vi "old LED STATUS for BLINKIN.vi"() -> ()   [LabVIEW 2023]
uses:
  ctrl defs/ctrl LED STATES.ctl
  <vilib>/Rock Robotics/WPI/DriverStation/WPI_DriverStationRobotMode2.ctl
  <vilib>/Rock Robotics/WPI/DriverStation/WPI_DriverStationAllianceInfo.ctl
  ctrl defs/ctrl LED PATTERNS.ctl
  Global INIT.vi
  Global stack names.vi
  <vilib>/Rock Robotics/Network Tables/NT Read Boolean.vi
  Global odometry.vi
panel:
  in  "ARMS LOCKED":T1=22 items=["<<Select a pattern>>", "Rainbow, Rainbow palette", "Rainbow, Party palette", "Rainbow, Ocean palette", "Rainbow, Lava palette", "Rainbow, Forest palette", "Rainbow with glitter", "Confetti", "Shot, Red", "Shot, Blue", "Shot, White", "Sinelon, Rainbow palette", "Sinelon, Party palette", "Sinelon, Ocean palette", "Sinelon, Lava palette", "Sinelon, Forest palette", "BPM, Rainbow palette", "BPM, Party palette", "BPM, Ocean palette", "BPM, Lava palette", "BPM, Forest palette", "Fire, Medium", "Fire, Large", "Twinkles, Rainbow palette", "Twinkles, Party palette", "Twinkles, Ocean palette", "Twinkles, Lava palette", "Twinkles, Forest palette", "Color Waves, Rainbow palette", "Color Waves, Party palette", "Color Waves, Ocean palette", "Color Waves, Lava palette", "Color Waves, Forest palette", "Larson Scanner, Red", "Larson Scanner, Gray", "Light Chase, Red", "Light Chase, Blue", "Light Chase, Gray", "Heartbeat, Red", "Heartbeat, Blue", "Heartbeat, White", "Heartbeat, Gray", "Breath, Red", "Breath, Blue", "Breath, Gray", "Strobe, Red", "Strobe, Blue", "Strobe, Gold", "Strobe, White", "Color 1: End to End Blend to Black", "Color 1: Larson Scanner", "Color 1: Light Chase", "Color 1: Heartbeat Slow", "Color 1: Heartbeat Medium", "Color 1: Heartbeat Fast", "Color 1: Breath Slow", "Color 1: Breath Fast", "Color 1: Shot", "Color 1: Strobe", "Color 2: End to End Blend to Black", "Color 2: Larson Scanner", "Color 2: Light Chase", "Color 2: Heartbeat Slow", "Color 2: Heartbeat Medium", "Color 2: Heartbeat Fast", "Color 2: Breath Slow", "Color 2: Breath Fast", "Color 2: Shot", "Color 2: Strobe", "Color 1/2: Sparkle, 1 on 2", "Color 1/2: Sparkle 2 on 1", "Color 1/2: Gradient", "Color 1/2: BPM", "Color 1/2: End to End Blend 1 to 2", "Color 1/2: End to End Blend 2 to 1", "Color 1/2: setup pattern", "Color 1/2: Twinkles", "Color 1/2: Color Waves", "Color 1/2: Sinelon", "Solid Hot Pink", "Solid Dark Red", "Solid Red", "Solid Red Orange", "Solid Orange", "Solid Gold", "Solid Yellow", "Solid Lawn Green", "Solid Lime", "Solid Dark Green", "Solid Green", "Solid Blue Green", "Solid Aqua", "Solid Sky Blue", "Solid Dark Blue", "Solid Blue", "Solid Blue Violet", "Solid Violet", "Solid White", "Solid Gray", "Solid Dark Gray", "Solid Black"]
  in  "PUKE":T1=79 items=["<<Select a pattern>>", "Rainbow, Rainbow palette", "Rainbow, Party palette", "Rainbow, Ocean palette", "Rainbow, Lava palette", "Rainbow, Forest palette", "Rainbow with glitter", "Confetti", "Shot, Red", "Shot, Blue", "Shot, White", "Sinelon, Rainbow palette", "Sinelon, Party palette", "Sinelon, Ocean palette", "Sinelon, Lava palette", "Sinelon, Forest palette", "BPM, Rainbow palette", "BPM, Party palette", "BPM, Ocean palette", "BPM, Lava palette", "BPM, Forest palette", "Fire, Medium", "Fire, Large", "Twinkles, Rainbow palette", "Twinkles, Party palette", "Twinkles, Ocean palette", "Twinkles, Lava palette", "Twinkles, Forest palette", "Color Waves, Rainbow palette", "Color Waves, Party palette", "Color Waves, Ocean palette", "Color Waves, Lava palette", "Color Waves, Forest palette", "Larson Scanner, Red", "Larson Scanner, Gray", "Light Chase, Red", "Light Chase, Blue", "Light Chase, Gray", "Heartbeat, Red", "Heartbeat, Blue", "Heartbeat, White", "Heartbeat, Gray", "Breath, Red", "Breath, Blue", "Breath, Gray", "Strobe, Red", "Strobe, Blue", "Strobe, Gold", "Strobe, White", "Color 1: End to End Blend to Black", "Color 1: Larson Scanner", "Color 1: Light Chase", "Color 1: Heartbeat Slow", "Color 1: Heartbeat Medium", "Color 1: Heartbeat Fast", "Color 1: Breath Slow", "Color 1: Breath Fast", "Color 1: Shot", "Color 1: Strobe", "Color 2: End to End Blend to Black", "Color 2: Larson Scanner", "Color 2: Light Chase", "Color 2: Heartbeat Slow", "Color 2: Heartbeat Medium", "Color 2: Heartbeat Fast", "Color 2: Breath Slow", "Color 2: Breath Fast", "Color 2: Shot", "Color 2: Strobe", "Color 1/2: Sparkle, 1 on 2", "Color 1/2: Sparkle 2 on 1", "Color 1/2: Gradient", "Color 1/2: BPM", "Color 1/2: End to End Blend 1 to 2", "Color 1/2: End to End Blend 2 to 1", "Color 1/2: setup pattern", "Color 1/2: Twinkles", "Color 1/2: Color Waves", "Color 1/2: Sinelon", "Solid Hot Pink", "Solid Dark Red", "Solid Red", "Solid Red Orange", "Solid Orange", "Solid Gold", "Solid Yellow", "Solid Lawn Green", "Solid Lime", "Solid Dark Green", "Solid Green", "Solid Blue Green", "Solid Aqua", "Solid Sky Blue", "Solid Dark Blue", "Solid Blue", "Solid Blue Violet", "Solid Violet", "Solid White", "Solid Gray", "Solid Dark Gray", "Solid Black"]
  in  "LOOKING for NOTE":T1=33 items=["<<Select a pattern>>", "Rainbow, Rainbow palette", "Rainbow, Party palette", "Rainbow, Ocean palette", "Rainbow, Lava palette", "Rainbow, Forest palette", "Rainbow with glitter", "Confetti", "Shot, Red", "Shot, Blue", "Shot, White", "Sinelon, Rainbow palette", "Sinelon, Party palette", "Sinelon, Ocean palette", "Sinelon, Lava palette", "Sinelon, Forest palette", "BPM, Rainbow palette", "BPM, Party palette", "BPM, Ocean palette", "BPM, Lava palette", "BPM, Forest palette", "Fire, Medium", "Fire, Large", "Twinkles, Rainbow palette", "Twinkles, Party palette", "Twinkles, Ocean palette", "Twinkles, Lava palette", "Twinkles, Forest palette", "Color Waves, Rainbow palette", "Color Waves, Party palette", "Color Waves, Ocean palette", "Color Waves, Lava palette", "Color Waves, Forest palette", "Larson Scanner, Red", "Larson Scanner, Gray", "Light Chase, Red", "Light Chase, Blue", "Light Chase, Gray", "Heartbeat, Red", "Heartbeat, Blue", "Heartbeat, White", "Heartbeat, Gray", "Breath, Red", "Breath, Blue", "Breath, Gray", "Strobe, Red", "Strobe, Blue", "Strobe, Gold", "Strobe, White", "Color 1: End to End Blend to Black", "Color 1: Larson Scanner", "Color 1: Light Chase", "Color 1: Heartbeat Slow", "Color 1: Heartbeat Medium", "Color 1: Heartbeat Fast", "Color 1: Breath Slow", "Color 1: Breath Fast", "Color 1: Shot", "Color 1: Strobe", "Color 2: End to End Blend to Black", "Color 2: Larson Scanner", "Color 2: Light Chase", "Color 2: Heartbeat Slow", "Color 2: Heartbeat Medium", "Color 2: Heartbeat Fast", "Color 2: Breath Slow", "Color 2: Breath Fast", "Color 2: Shot", "Color 2: Strobe", "Color 1/2: Sparkle, 1 on 2", "Color 1/2: Sparkle 2 on 1", "Color 1/2: Gradient", "Color 1/2: BPM", "Color 1/2: End to End Blend 1 to 2", "Color 1/2: End to End Blend 2 to 1", "Color 1/2: setup pattern", "Color 1/2: Twinkles", "Color 1/2: Color Waves", "Color 1/2: Sinelon", "Solid Hot Pink", "Solid Dark Red", "Solid Red", "Solid Red Orange", "Solid Orange", "Solid Gold", "Solid Yellow", "Solid Lawn Green", "Solid Lime", "Solid Dark Green", "Solid Green", "Solid Blue Green", "Solid Aqua", "Solid Sky Blue", "Solid Dark Blue", "Solid Blue", "Solid Blue Violet", "Solid Violet", "Solid White", "Solid Gray", "Solid Dark Gray", "Solid Black"]
  in  "NOTE LOADED":T1=89 items=["<<Select a pattern>>", "Rainbow, Rainbow palette", "Rainbow, Party palette", "Rainbow, Ocean palette", "Rainbow, Lava palette", "Rainbow, Forest palette", "Rainbow with glitter", "Confetti", "Shot, Red", "Shot, Blue", "Shot, White", "Sinelon, Rainbow palette", "Sinelon, Party palette", "Sinelon, Ocean palette", "Sinelon, Lava palette", "Sinelon, Forest palette", "BPM, Rainbow palette", "BPM, Party palette", "BPM, Ocean palette", "BPM, Lava palette", "BPM, Forest palette", "Fire, Medium", "Fire, Large", "Twinkles, Rainbow palette", "Twinkles, Party palette", "Twinkles, Ocean palette", "Twinkles, Lava palette", "Twinkles, Forest palette", "Color Waves, Rainbow palette", "Color Waves, Party palette", "Color Waves, Ocean palette", "Color Waves, Lava palette", "Color Waves, Forest palette", "Larson Scanner, Red", "Larson Scanner, Gray", "Light Chase, Red", "Light Chase, Blue", "Light Chase, Gray", "Heartbeat, Red", "Heartbeat, Blue", "Heartbeat, White", "Heartbeat, Gray", "Breath, Red", "Breath, Blue", "Breath, Gray", "Strobe, Red", "Strobe, Blue", "Strobe, Gold", "Strobe, White", "Color 1: End to End Blend to Black", "Color 1: Larson Scanner", "Color 1: Light Chase", "Color 1: Heartbeat Slow", "Color 1: Heartbeat Medium", "Color 1: Heartbeat Fast", "Color 1: Breath Slow", "Color 1: Breath Fast", "Color 1: Shot", "Color 1: Strobe", "Color 2: End to End Blend to Black", "Color 2: Larson Scanner", "Color 2: Light Chase", "Color 2: Heartbeat Slow", "Color 2: Heartbeat Medium", "Color 2: Heartbeat Fast", "Color 2: Breath Slow", "Color 2: Breath Fast", "Color 2: Shot", "Color 2: Strobe", "Color 1/2: Sparkle, 1 on 2", "Color 1/2: Sparkle 2 on 1", "Color 1/2: Gradient", "Color 1/2: BPM", "Color 1/2: End to End Blend 1 to 2", "Color 1/2: End to End Blend 2 to 1", "Color 1/2: setup pattern", "Color 1/2: Twinkles", "Color 1/2: Color Waves", "Color 1/2: Sinelon", "Solid Hot Pink", "Solid Dark Red", "Solid Red", "Solid Red Orange", "Solid Orange", "Solid Gold", "Solid Yellow", "Solid Lawn Green", "Solid Lime", "Solid Dark Green", "Solid Green", "Solid Blue Green", "Solid Aqua", "Solid Sky Blue", "Solid Dark Blue", "Solid Blue", "Solid Blue Violet", "Solid Violet", "Solid White", "Solid Gray", "Solid Dark Gray", "Solid Black"]
  in  "END GAME 2":T1=94 items=["<<Select a pattern>>", "Rainbow, Rainbow palette", "Rainbow, Party palette", "Rainbow, Ocean palette", "Rainbow, Lava palette", "Rainbow, Forest palette", "Rainbow with glitter", "Confetti", "Shot, Red", "Shot, Blue", "Shot, White", "Sinelon, Rainbow palette", "Sinelon, Party palette", "Sinelon, Ocean palette", "Sinelon, Lava palette", "Sinelon, Forest palette", "BPM, Rainbow palette", "BPM, Party palette", "BPM, Ocean palette", "BPM, Lava palette", "BPM, Forest palette", "Fire, Medium", "Fire, Large", "Twinkles, Rainbow palette", "Twinkles, Party palette", "Twinkles, Ocean palette", "Twinkles, Lava palette", "Twinkles, Forest palette", "Color Waves, Rainbow palette", "Color Waves, Party palette", "Color Waves, Ocean palette", "Color Waves, Lava palette", "Color Waves, Forest palette", "Larson Scanner, Red", "Larson Scanner, Gray", "Light Chase, Red", "Light Chase, Blue", "Light Chase, Gray", "Heartbeat, Red", "Heartbeat, Blue", "Heartbeat, White", "Heartbeat, Gray", "Breath, Red", "Breath, Blue", "Breath, Gray", "Strobe, Red", "Strobe, Blue", "Strobe, Gold", "Strobe, White", "Color 1: End to End Blend to Black", "Color 1: Larson Scanner", "Color 1: Light Chase", "Color 1: Heartbeat Slow", "Color 1: Heartbeat Medium", "Color 1: Heartbeat Fast", "Color 1: Breath Slow", "Color 1: Breath Fast", "Color 1: Shot", "Color 1: Strobe", "Color 2: End to End Blend to Black", "Color 2: Larson Scanner", "Color 2: Light Chase", "Color 2: Heartbeat Slow", "Color 2: Heartbeat Medium", "Color 2: Heartbeat Fast", "Color 2: Breath Slow", "Color 2: Breath Fast", "Color 2: Shot", "Color 2: Strobe", "Color 1/2: Sparkle, 1 on 2", "Color 1/2: Sparkle 2 on 1", "Color 1/2: Gradient", "Color 1/2: BPM", "Color 1/2: End to End Blend 1 to 2", "Color 1/2: End to End Blend 2 to 1", "Color 1/2: setup pattern", "Color 1/2: Twinkles", "Color 1/2: Color Waves", "Color 1/2: Sinelon", "Solid Hot Pink", "Solid Dark Red", "Solid Red", "Solid Red Orange", "Solid Orange", "Solid Gold", "Solid Yellow", "Solid Lawn Green", "Solid Lime", "Solid Dark Green", "Solid Green", "Solid Blue Green", "Solid Aqua", "Solid Sky Blue", "Solid Dark Blue", "Solid Blue", "Solid Blue Violet", "Solid Violet", "Solid White", "Solid Gray", "Solid Dark Gray", "Solid Black"]
  in  "END GAME 1":T1=85 items=["<<Select a pattern>>", "Rainbow, Rainbow palette", "Rainbow, Party palette", "Rainbow, Ocean palette", "Rainbow, Lava palette", "Rainbow, Forest palette", "Rainbow with glitter", "Confetti", "Shot, Red", "Shot, Blue", "Shot, White", "Sinelon, Rainbow palette", "Sinelon, Party palette", "Sinelon, Ocean palette", "Sinelon, Lava palette", "Sinelon, Forest palette", "BPM, Rainbow palette", "BPM, Party palette", "BPM, Ocean palette", "BPM, Lava palette", "BPM, Forest palette", "Fire, Medium", "Fire, Large", "Twinkles, Rainbow palette", "Twinkles, Party palette", "Twinkles, Ocean palette", "Twinkles, Lava palette", "Twinkles, Forest palette", "Color Waves, Rainbow palette", "Color Waves, Party palette", "Color Waves, Ocean palette", "Color Waves, Lava palette", "Color Waves, Forest palette", "Larson Scanner, Red", "Larson Scanner, Gray", "Light Chase, Red", "Light Chase, Blue", "Light Chase, Gray", "Heartbeat, Red", "Heartbeat, Blue", "Heartbeat, White", "Heartbeat, Gray", "Breath, Red", "Breath, Blue", "Breath, Gray", "Strobe, Red", "Strobe, Blue", "Strobe, Gold", "Strobe, White", "Color 1: End to End Blend to Black", "Color 1: Larson Scanner", "Color 1: Light Chase", "Color 1: Heartbeat Slow", "Color 1: Heartbeat Medium", "Color 1: Heartbeat Fast", "Color 1: Breath Slow", "Color 1: Breath Fast", "Color 1: Shot", "Color 1: Strobe", "Color 2: End to End Blend to Black", "Color 2: Larson Scanner", "Color 2: Light Chase", "Color 2: Heartbeat Slow", "Color 2: Heartbeat Medium", "Color 2: Heartbeat Fast", "Color 2: Breath Slow", "Color 2: Breath Fast", "Color 2: Shot", "Color 2: Strobe", "Color 1/2: Sparkle, 1 on 2", "Color 1/2: Sparkle 2 on 1", "Color 1/2: Gradient", "Color 1/2: BPM", "Color 1/2: End to End Blend 1 to 2", "Color 1/2: End to End Blend 2 to 1", "Color 1/2: setup pattern", "Color 1/2: Twinkles", "Color 1/2: Color Waves", "Color 1/2: Sinelon", "Solid Hot Pink", "Solid Dark Red", "Solid Red", "Solid Red Orange", "Solid Orange", "Solid Gold", "Solid Yellow", "Solid Lawn Green", "Solid Lime", "Solid Dark Green", "Solid Green", "Solid Blue Green", "Solid Aqua", "Solid Sky Blue", "Solid Dark Blue", "Solid Blue", "Solid Blue Violet", "Solid Violet", "Solid White", "Solid Gray", "Solid Dark Gray", "Solid Black"]
  in  "LOW BATT":T1=45 items=["<<Select a pattern>>", "Rainbow, Rainbow palette", "Rainbow, Party palette", "Rainbow, Ocean palette", "Rainbow, Lava palette", "Rainbow, Forest palette", "Rainbow with glitter", "Confetti", "Shot, Red", "Shot, Blue", "Shot, White", "Sinelon, Rainbow palette", "Sinelon, Party palette", "Sinelon, Ocean palette", "Sinelon, Lava palette", "Sinelon, Forest palette", "BPM, Rainbow palette", "BPM, Party palette", "BPM, Ocean palette", "BPM, Lava palette", "BPM, Forest palette", "Fire, Medium", "Fire, Large", "Twinkles, Rainbow palette", "Twinkles, Party palette", "Twinkles, Ocean palette", "Twinkles, Lava palette", "Twinkles, Forest palette", "Color Waves, Rainbow palette", "Color Waves, Party palette", "Color Waves, Ocean palette", "Color Waves, Lava palette", "Color Waves, Forest palette", "Larson Scanner, Red", "Larson Scanner, Gray", "Light Chase, Red", "Light Chase, Blue", "Light Chase, Gray", "Heartbeat, Red", "Heartbeat, Blue", "Heartbeat, White", "Heartbeat, Gray", "Breath, Red", "Breath, Blue", "Breath, Gray", "Strobe, Red", "Strobe, Blue", "Strobe, Gold", "Strobe, White", "Color 1: End to End Blend to Black", "Color 1: Larson Scanner", "Color 1: Light Chase", "Color 1: Heartbeat Slow", "Color 1: Heartbeat Medium", "Color 1: Heartbeat Fast", "Color 1: Breath Slow", "Color 1: Breath Fast", "Color 1: Shot", "Color 1: Strobe", "Color 2: End to End Blend to Black", "Color 2: Larson Scanner", "Color 2: Light Chase", "Color 2: Heartbeat Slow", "Color 2: Heartbeat Medium", "Color 2: Heartbeat Fast", "Color 2: Breath Slow", "Color 2: Breath Fast", "Color 2: Shot", "Color 2: Strobe", "Color 1/2: Sparkle, 1 on 2", "Color 1/2: Sparkle 2 on 1", "Color 1/2: Gradient", "Color 1/2: BPM", "Color 1/2: End to End Blend 1 to 2", "Color 1/2: End to End Blend 2 to 1", "Color 1/2: setup pattern", "Color 1/2: Twinkles", "Color 1/2: Color Waves", "Color 1/2: Sinelon", "Solid Hot Pink", "Solid Dark Red", "Solid Red", "Solid Red Orange", "Solid Orange", "Solid Gold", "Solid Yellow", "Solid Lawn Green", "Solid Lime", "Solid Dark Green", "Solid Green", "Solid Blue Green", "Solid Aqua", "Solid Sky Blue", "Solid Dark Blue", "Solid Blue", "Solid Blue Violet", "Solid Violet", "Solid White", "Solid Gray", "Solid Dark Gray", "Solid Black"]
  in  "SELECT  AMP":T1=47 items=["<<Select a pattern>>", "Rainbow, Rainbow palette", "Rainbow, Party palette", "Rainbow, Ocean palette", "Rainbow, Lava palette", "Rainbow, Forest palette", "Rainbow with glitter", "Confetti", "Shot, Red", "Shot, Blue", "Shot, White", "Sinelon, Rainbow palette", "Sinelon, Party palette", "Sinelon, Ocean palette", "Sinelon, Lava palette", "Sinelon, Forest palette", "BPM, Rainbow palette", "BPM, Party palette", "BPM, Ocean palette", "BPM, Lava palette", "BPM, Forest palette", "Fire, Medium", "Fire, Large", "Twinkles, Rainbow palette", "Twinkles, Party palette", "Twinkles, Ocean palette", "Twinkles, Lava palette", "Twinkles, Forest palette", "Color Waves, Rainbow palette", "Color Waves, Party palette", "Color Waves, Ocean palette", "Color Waves, Lava palette", "Color Waves, Forest palette", "Larson Scanner, Red", "Larson Scanner, Gray", "Light Chase, Red", "Light Chase, Blue", "Light Chase, Gray", "Heartbeat, Red", "Heartbeat, Blue", "Heartbeat, White", "Heartbeat, Gray", "Breath, Red", "Breath, Blue", "Breath, Gray", "Strobe, Red", "Strobe, Blue", "Strobe, Gold", "Strobe, White", "Color 1: End to End Blend to Black", "Color 1: Larson Scanner", "Color 1: Light Chase", "Color 1: Heartbeat Slow", "Color 1: Heartbeat Medium", "Color 1: Heartbeat Fast", "Color 1: Breath Slow", "Color 1: Breath Fast", "Color 1: Shot", "Color 1: Strobe", "Color 2: End to End Blend to Black", "Color 2: Larson Scanner", "Color 2: Light Chase", "Color 2: Heartbeat Slow", "Color 2: Heartbeat Medium", "Color 2: Heartbeat Fast", "Color 2: Breath Slow", "Color 2: Breath Fast", "Color 2: Shot", "Color 2: Strobe", "Color 1/2: Sparkle, 1 on 2", "Color 1/2: Sparkle 2 on 1", "Color 1/2: Gradient", "Color 1/2: BPM", "Color 1/2: End to End Blend 1 to 2", "Color 1/2: End to End Blend 2 to 1", "Color 1/2: setup pattern", "Color 1/2: Twinkles", "Color 1/2: Color Waves", "Color 1/2: Sinelon", "Solid Hot Pink", "Solid Dark Red", "Solid Red", "Solid Red Orange", "Solid Orange", "Solid Gold", "Solid Yellow", "Solid Lawn Green", "Solid Lime", "Solid Dark Green", "Solid Green", "Solid Blue Green", "Solid Aqua", "Solid Sky Blue", "Solid Dark Blue", "Solid Blue", "Solid Blue Violet", "Solid Violet", "Solid White", "Solid Gray", "Solid Dark Gray", "Solid Black"]
  in  "FIRE":T1=84 items=["<<Select a pattern>>", "Rainbow, Rainbow palette", "Rainbow, Party palette", "Rainbow, Ocean palette", "Rainbow, Lava palette", "Rainbow, Forest palette", "Rainbow with glitter", "Confetti", "Shot, Red", "Shot, Blue", "Shot, White", "Sinelon, Rainbow palette", "Sinelon, Party palette", "Sinelon, Ocean palette", "Sinelon, Lava palette", "Sinelon, Forest palette", "BPM, Rainbow palette", "BPM, Party palette", "BPM, Ocean palette", "BPM, Lava palette", "BPM, Forest palette", "Fire, Medium", "Fire, Large", "Twinkles, Rainbow palette", "Twinkles, Party palette", "Twinkles, Ocean palette", "Twinkles, Lava palette", "Twinkles, Forest palette", "Color Waves, Rainbow palette", "Color Waves, Party palette", "Color Waves, Ocean palette", "Color Waves, Lava palette", "Color Waves, Forest palette", "Larson Scanner, Red", "Larson Scanner, Gray", "Light Chase, Red", "Light Chase, Blue", "Light Chase, Gray", "Heartbeat, Red", "Heartbeat, Blue", "Heartbeat, White", "Heartbeat, Gray", "Breath, Red", "Breath, Blue", "Breath, Gray", "Strobe, Red", "Strobe, Blue", "Strobe, Gold", "Strobe, White", "Color 1: End to End Blend to Black", "Color 1: Larson Scanner", "Color 1: Light Chase", "Color 1: Heartbeat Slow", "Color 1: Heartbeat Medium", "Color 1: Heartbeat Fast", "Color 1: Breath Slow", "Color 1: Breath Fast", "Color 1: Shot", "Color 1: Strobe", "Color 2: End to End Blend to Black", "Color 2: Larson Scanner", "Color 2: Light Chase", "Color 2: Heartbeat Slow", "Color 2: Heartbeat Medium", "Color 2: Heartbeat Fast", "Color 2: Breath Slow", "Color 2: Breath Fast", "Color 2: Shot", "Color 2: Strobe", "Color 1/2: Sparkle, 1 on 2", "Color 1/2: Sparkle 2 on 1", "Color 1/2: Gradient", "Color 1/2: BPM", "Color 1/2: End to End Blend 1 to 2", "Color 1/2: End to End Blend 2 to 1", "Color 1/2: setup pattern", "Color 1/2: Twinkles", "Color 1/2: Color Waves", "Color 1/2: Sinelon", "Solid Hot Pink", "Solid Dark Red", "Solid Red", "Solid Red Orange", "Solid Orange", "Solid Gold", "Solid Yellow", "Solid Lawn Green", "Solid Lime", "Solid Dark Green", "Solid Green", "Solid Blue Green", "Solid Aqua", "Solid Sky Blue", "Solid Dark Blue", "Solid Blue", "Solid Blue Violet", "Solid Violet", "Solid White", "Solid Gray", "Solid Dark Gray", "Solid Black"]
  in  "DEFAULT":T1=75 items=["<<Select a pattern>>", "Rainbow, Rainbow palette", "Rainbow, Party palette", "Rainbow, Ocean palette", "Rainbow, Lava palette", "Rainbow, Forest palette", "Rainbow with glitter", "Confetti", "Shot, Red", "Shot, Blue", "Shot, White", "Sinelon, Rainbow palette", "Sinelon, Party palette", "Sinelon, Ocean palette", "Sinelon, Lava palette", "Sinelon, Forest palette", "BPM, Rainbow palette", "BPM, Party palette", "BPM, Ocean palette", "BPM, Lava palette", "BPM, Forest palette", "Fire, Medium", "Fire, Large", "Twinkles, Rainbow palette", "Twinkles, Party palette", "Twinkles, Ocean palette", "Twinkles, Lava palette", "Twinkles, Forest palette", "Color Waves, Rainbow palette", "Color Waves, Party palette", "Color Waves, Ocean palette", "Color Waves, Lava palette", "Color Waves, Forest palette", "Larson Scanner, Red", "Larson Scanner, Gray", "Light Chase, Red", "Light Chase, Blue", "Light Chase, Gray", "Heartbeat, Red", "Heartbeat, Blue", "Heartbeat, White", "Heartbeat, Gray", "Breath, Red", "Breath, Blue", "Breath, Gray", "Strobe, Red", "Strobe, Blue", "Strobe, Gold", "Strobe, White", "Color 1: End to End Blend to Black", "Color 1: Larson Scanner", "Color 1: Light Chase", "Color 1: Heartbeat Slow", "Color 1: Heartbeat Medium", "Color 1: Heartbeat Fast", "Color 1: Breath Slow", "Color 1: Breath Fast", "Color 1: Shot", "Color 1: Strobe", "Color 2: End to End Blend to Black", "Color 2: Larson Scanner", "Color 2: Light Chase", "Color 2: Heartbeat Slow", "Color 2: Heartbeat Medium", "Color 2: Heartbeat Fast", "Color 2: Breath Slow", "Color 2: Breath Fast", "Color 2: Shot", "Color 2: Strobe", "Color 1/2: Sparkle, 1 on 2", "Color 1/2: Sparkle 2 on 1", "Color 1/2: Gradient", "Color 1/2: BPM", "Color 1/2: End to End Blend 1 to 2", "Color 1/2: End to End Blend 2 to 1", "Color 1/2: setup pattern", "Color 1/2: Twinkles", "Color 1/2: Color Waves", "Color 1/2: Sinelon", "Solid Hot Pink", "Solid Dark Red", "Solid Red", "Solid Red Orange", "Solid Orange", "Solid Gold", "Solid Yellow", "Solid Lawn Green", "Solid Lime", "Solid Dark Green", "Solid Green", "Solid Blue Green", "Solid Aqua", "Solid Sky Blue", "Solid Dark Blue", "Solid Blue", "Solid Blue Violet", "Solid Violet", "Solid White", "Solid Gray", "Solid Dark Gray", "Solid Black"]
  out "Teleop indicators":T2
  out "Motor Output":dbl=0.49
  out "String":string="1 - Rainbow, Rainbow Palette\n2 - Rainbow, Party Palette\n3 - Rainbow, Ocean Palette\n4 - Rainbow, Lave Palette\n5 - Rainbow, Forest Palette\n6 - Rainbow with Glitter\n7 - Confetti\n8 - Shot, Red\n9 - Shot, Blue\n10 - Shot, White\n11 - Sinelon, Rainbow Palette\n12 - Sinelon, Party Palette\n13 - Sinelon, Ocean Palette\n14 - Sinelon, Lava Palette\n15 - Sinelon, Forest Palette\n16 - Beats per Minute, Rainbow Palette\n17 - Beats per Minute, Party Palette\n18 - Beats per Minute, Ocean Palette\n19 - Beats per Minute, Lava Palette\n20 - Beats per Minute, Forest Palette\n21 - Fire, Medium\n22 - Fire, Large\n23 - Twinkles, Rainbow Palette\n24 - Twinkles, Party Palette\n25 - Twinkles, Ocean Palette\n26 - Twinkles, Lava Palette\n27 - Twinkles, Forest Palette\n28 - Color Waves, Rainbow Palette\n29 - Color Waves, Party Palette\n30 - Color Waves, Ocean Palette\n31 - Color Waves, Lava Palette\n32 - Color Waves, Forest Palette\n33 - Larson Scanner, Red\n34 - Larson Scanner, Gray\n35 - Light Chase, Red\n36 - Light Chase, Blue\n37 - Light Chase, Gray\n38 - Heartbeat, Red\n39 - Heartbeat, Blue\n40 - Heartbeat, White\n41 - Heartbeat, Gray\n42 - Breath, Red\n43 - Breath, Blue\n44 - Breath, Gray\n45 - Strobe, Red\n46 - Strobe, Blue\n47 - Strobe, Gold\n48 - Strobe, White\n49 - Color 1: End to End Blend to Black\n50 - Color 1: Larson Scanner\n51 - Color 1: Light Chase\n52 - Color 1: Heartbeat Slow\n53 - Color 1: Heartbeat Medium\n54 - Color 1: Heartbeat Fast\n55 - Color 1: Breath Slow\n56 - Color 1: Breath Fast\n57 - Color 1: Shot\n58 - Color 1: Strobe\n59 - Color 2: End to End Blend to Black\n60 - Color 2: Larson Scanner\n61 - Color 2: Light Chase\n62 - Color 2: Heartbeat Slow\n63 - Color 2: Heartbeat Medium\n64 - Color 2: Heartbeat Fast\n65 - Color 2: Breath Slow\n66 - Color 2: Breath Fast\n67 - Color 2: Shot\n68 - Color 2: Strobe\n69 - Color 1/2: Sparkle, Color 1 on Color 2\n70 - Color 1/2: Sparkle, Color 2 on Color 1\n71 - Color 1/2: Color Gradient, Color 1 and 2\n72 - Color 1/2: Beats per Minute, Color 1 and 2\n73 - Color 1/2: End to End Blend, Color 1 to 2\n74 - Color 1/2: End to End Blend\n75 - Color 1/2:  no blending (Setup Pattern)\n76 - Color 1/2: Twinkles\n77 - Color 1/2: Color Waves\n78 - Color 1/2: Sinelon\n79 - Solid Hot Pink\n80 - Solid Dark red\n81 - Solid Red\n82 - Solid Red Orange\n83 - Solid Orange\n84 - Solid Gold\n85 - Solid Yellow\n86 - Solid Lawn Green\n87 - Solid Lime\n88 - Solid Dark Green\n89 - Solid Green\n90 - Solid Blue Green\n91 - Solid Aqua\n92 - Solid Sky Blue\n93 - Solid Dark Blue\n94 - Solid Blue\n95 - Solid Blue Violet\n96 - Solid Violet\n97 - Solid White\n98 - Solid Gray\n99 - Solid Dark Gray\n100 - Solid Black\n"
  out "SPARK value":dbl=0.49
  out "pattern\nindex":u16=75
  out "PULSE value":dbl=1745.0
  in  "pattern":T1=39 items=["<<Select a pattern>>", "Rainbow, Rainbow palette", "Rainbow, Party palette", "Rainbow, Ocean palette", "Rainbow, Lava palette", "Rainbow, Forest palette", "Rainbow with glitter", "Confetti", "Shot, Red", "Shot, Blue", "Shot, White", "Sinelon, Rainbow palette", "Sinelon, Party palette", "Sinelon, Ocean palette", "Sinelon, Lava palette", "Sinelon, Forest palette", "BPM, Rainbow palette", "BPM, Party palette", "BPM, Ocean palette", "BPM, Lava palette", "BPM, Forest palette", "Fire, Medium", "Fire, Large", "Twinkles, Rainbow palette", "Twinkles, Party palette", "Twinkles, Ocean palette", "Twinkles, Lava palette", "Twinkles, Forest palette", "Color Waves, Rainbow palette", "Color Waves, Party palette", "Color Waves, Ocean palette", "Color Waves, Lava palette", "Color Waves, Forest palette", "Larson Scanner, Red", "Larson Scanner, Gray", "Light Chase, Red", "Light Chase, Blue", "Light Chase, Gray", "Heartbeat, Red", "Heartbeat, Blue", "Heartbeat, White", "Heartbeat, Gray", "Breath, Red", "Breath, Blue", "Breath, Gray", "Strobe, Red", "Strobe, Blue", "Strobe, Gold", "Strobe, White", "Color 1: End to End Blend to Black", "Color 1: Larson Scanner", "Color 1: Light Chase", "Color 1: Heartbeat Slow", "Color 1: Heartbeat Medium", "Color 1: Heartbeat Fast", "Color 1: Breath Slow", "Color 1: Breath Fast", "Color 1: Shot", "Color 1: Strobe", "Color 2: End to End Blend to Black", "Color 2: Larson Scanner", "Color 2: Light Chase", "Color 2: Heartbeat Slow", "Color 2: Heartbeat Medium", "Color 2: Heartbeat Fast", "Color 2: Breath Slow", "Color 2: Breath Fast", "Color 2: Shot", "Color 2: Strobe", "Color 1/2: Sparkle, 1 on 2", "Color 1/2: Sparkle 2 on 1", "Color 1/2: Gradient", "Color 1/2: BPM", "Color 1/2: End to End Blend 1 to 2", "Color 1/2: End to End Blend 2 to 1", "Color 1/2: setup pattern", "Color 1/2: Twinkles", "Color 1/2: Color Waves", "Color 1/2: Sinelon", "Solid Hot Pink", "Solid Dark Red", "Solid Red", "Solid Red Orange", "Solid Orange", "Solid Gold", "Solid Yellow", "Solid Lawn Green", "Solid Lime", "Solid Dark Green", "Solid Green", "Solid Blue Green", "Solid Aqua", "Solid Sky Blue", "Solid Dark Blue", "Solid Blue", "Solid Blue Violet", "Solid Violet", "Solid White", "Solid Gray", "Solid Dark Gray", "Solid Black"]
  in  "manual\noveride":bool
  out "Alliance":T3
  out "Robot Mode":T4=enum."Teleop Enabled"
  out "Match Time(s)":sgl=-1.0
  out "LED state":T5=enum."WRITE LED VALUE"
  out "error out":errorcluster
  in  "error in (no error)":errorcluster
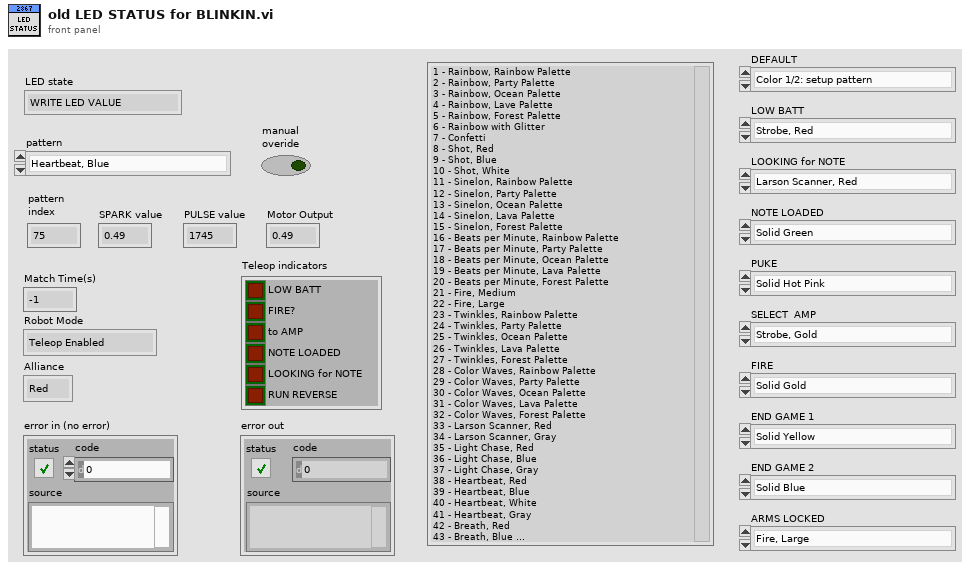
[diagram p1: front panel]
types:
  T1 = typedef "ctrl LED PATTERNS.ctl" = u16
  T2 = cluster{"LOW BATT":bool, "FIRE?":bool, "to AMP":bool, "NOTE LOADED":bool, "LOOKING for NOTE":bool, "RUN REVERSE":bool}
  T3 = typedef "WPI_DriverStationAllianceInfo.ctl" = enum16{"Red", "Blue", "Invalid"}
  T4 = typedef "WPI_DriverStationRobotMode2.ctl" = enum16{"Autonomous Disabled", "Autonomous Enabled", "Teleop Disabled", "Teleop Enabled", "Disconnected", "Finish", "Test Disabled", "Test Enabled", "Emergency Stopped"}
  T5 = typedef "ctrl LED STATES.ctl" = enum16{"STANDBY", "END GAME 1", "END GAME 2", "NOTE is LOADED", "LOOKING for NOTE", "PUKE", "FIRE", "SHOOT AMP", "EXTENDING ARMS", "RETRACTING ARMS", "ARMS LOCKED", "LOW BATTERY", "WRITE LED VALUE", "DEFAULT PATTERN"}
  T6 = typedef "ctrl LED init.ctl" = cluster{"PWM Channel":T7, "refnum name":string, "#LEDS":T8, "initial output":dbl, "stack name":string, "Installed?":bool, "pattern":T1}
  T7 = typedef "FPGA_DIOPWMChannel.ctl" = enum8{"PWM 0", "PWM 1", "PWM 2", "PWM 3", "PWM 4", "PWM 5", "PWM 6", "PWM 7", "PWM 8", "PWM 9", "PWM MXP 0", "PWM MXP 1", "PWM MXP 2", "PWM MXP 3", "PWM MXP 4", "PWM MXP 5", "PWM MXP 6", "PWM MXP 7", "PWM MXP 8", "PWM MXP 9", "Invalid"}
  T8 = typedef "ctrl number of LEDs.ctl" = u16
  T9 = typedef "WPI_MotorControlDeviceRef.ctl" = cluster{"DeviceStatus":errorcluster, "Type":T10, "PWM":cluster{"PWM Channel":T7, "DeadBand":T11}, "CAN":cluster{"Device Number":u8, "SetOutput VI Ref":variant, "GetOutput VI Ref":variant, "Enable VI Ref":variant, "Disable VI Ref":variant, "Data":variant}, "Invert":bool, "DIO PWM":cluster{"PWM \"Enable\" Channel":T7, "DIOChannel":T12, "PWM Rate":dbl}}
  T10 = typedef "WPI_MotorControlType.ctl" = enum16{"PWM", "CAN", "DIO PWM"}
  T11 = typedef "WPI_PWMDeadband.ctl" = cluster{"Name":string, "maxPositivePwm":i32, "minPositivePwm":i32, "centerPwm":i32, "maxNegativePwm":i32, "minNegativePwm":i32, "angularRange":u16}
  T12 = typedef "FPGA_DIOChannel.ctl" = enum8{"DIO 0", "DIO 1", "DIO 2", "DIO 3", "DIO 4", "DIO 5", "DIO 6", "DIO 7", "DIO 8", "DIO 9", "DIO MXP 0", "DIO MXP 1", "DIO MXP 2", "DIO MXP 3", "DIO MXP 4", "DIO MXP 5", "DIO MXP 6", "DIO MXP 7", "DIO MXP 8", "DIO MXP 9", "DIO MXP 10", "DIO MXP 11", "DIO MXP 12", "DIO MXP 13", "DIO MXP 14", "DIO MXP 15", "SPI Port CS1", "SPI Port CS2", "SPI Port CS3", "SPI Port MISO", "SPI Port MOSI", "Invalid"}
  T13 = typedef "ctrl stack - INTAKE SHOOTER.ctl" = cluster{"INTAKE STATE":string, "RUN INTAKE?":string, "RUN REVERSE?":string, "NOTE LOADED?":string, "SHOOTER STATE":string, "SHOOTER FIRE?":string, "SHOOT AMP?":string, "EXTEND FLAP?":string, "LOOKING for NOTE":string, "OVERIDE NOTE CHECK":string}
  T14 = cluster{"Battery Voltage Fault":bool, "Hardware Fault":bool, "CAN Warning Fault":bool, "Temperature Fault":bool}
  T15 = cluster{"Brownout":bool, "CAN Warning":bool, "Can Bus Off":bool, "Hardware Fault":bool, "Firmware Fault":bool, "CH20 Brownout":bool, "CH21 Brownout":bool, "CH22 Brownout":bool, "CH23 Brownout":bool, "Has Reset":bool}
  T16 = cluster{"LEFT ARM":cluster{"VBus%":dbl, "LOCK?":bool, "LOCKED":bool}, "RIGHT ARM":cluster{"VBus%":dbl, "LOCK?":bool, "LOCKED":bool}}
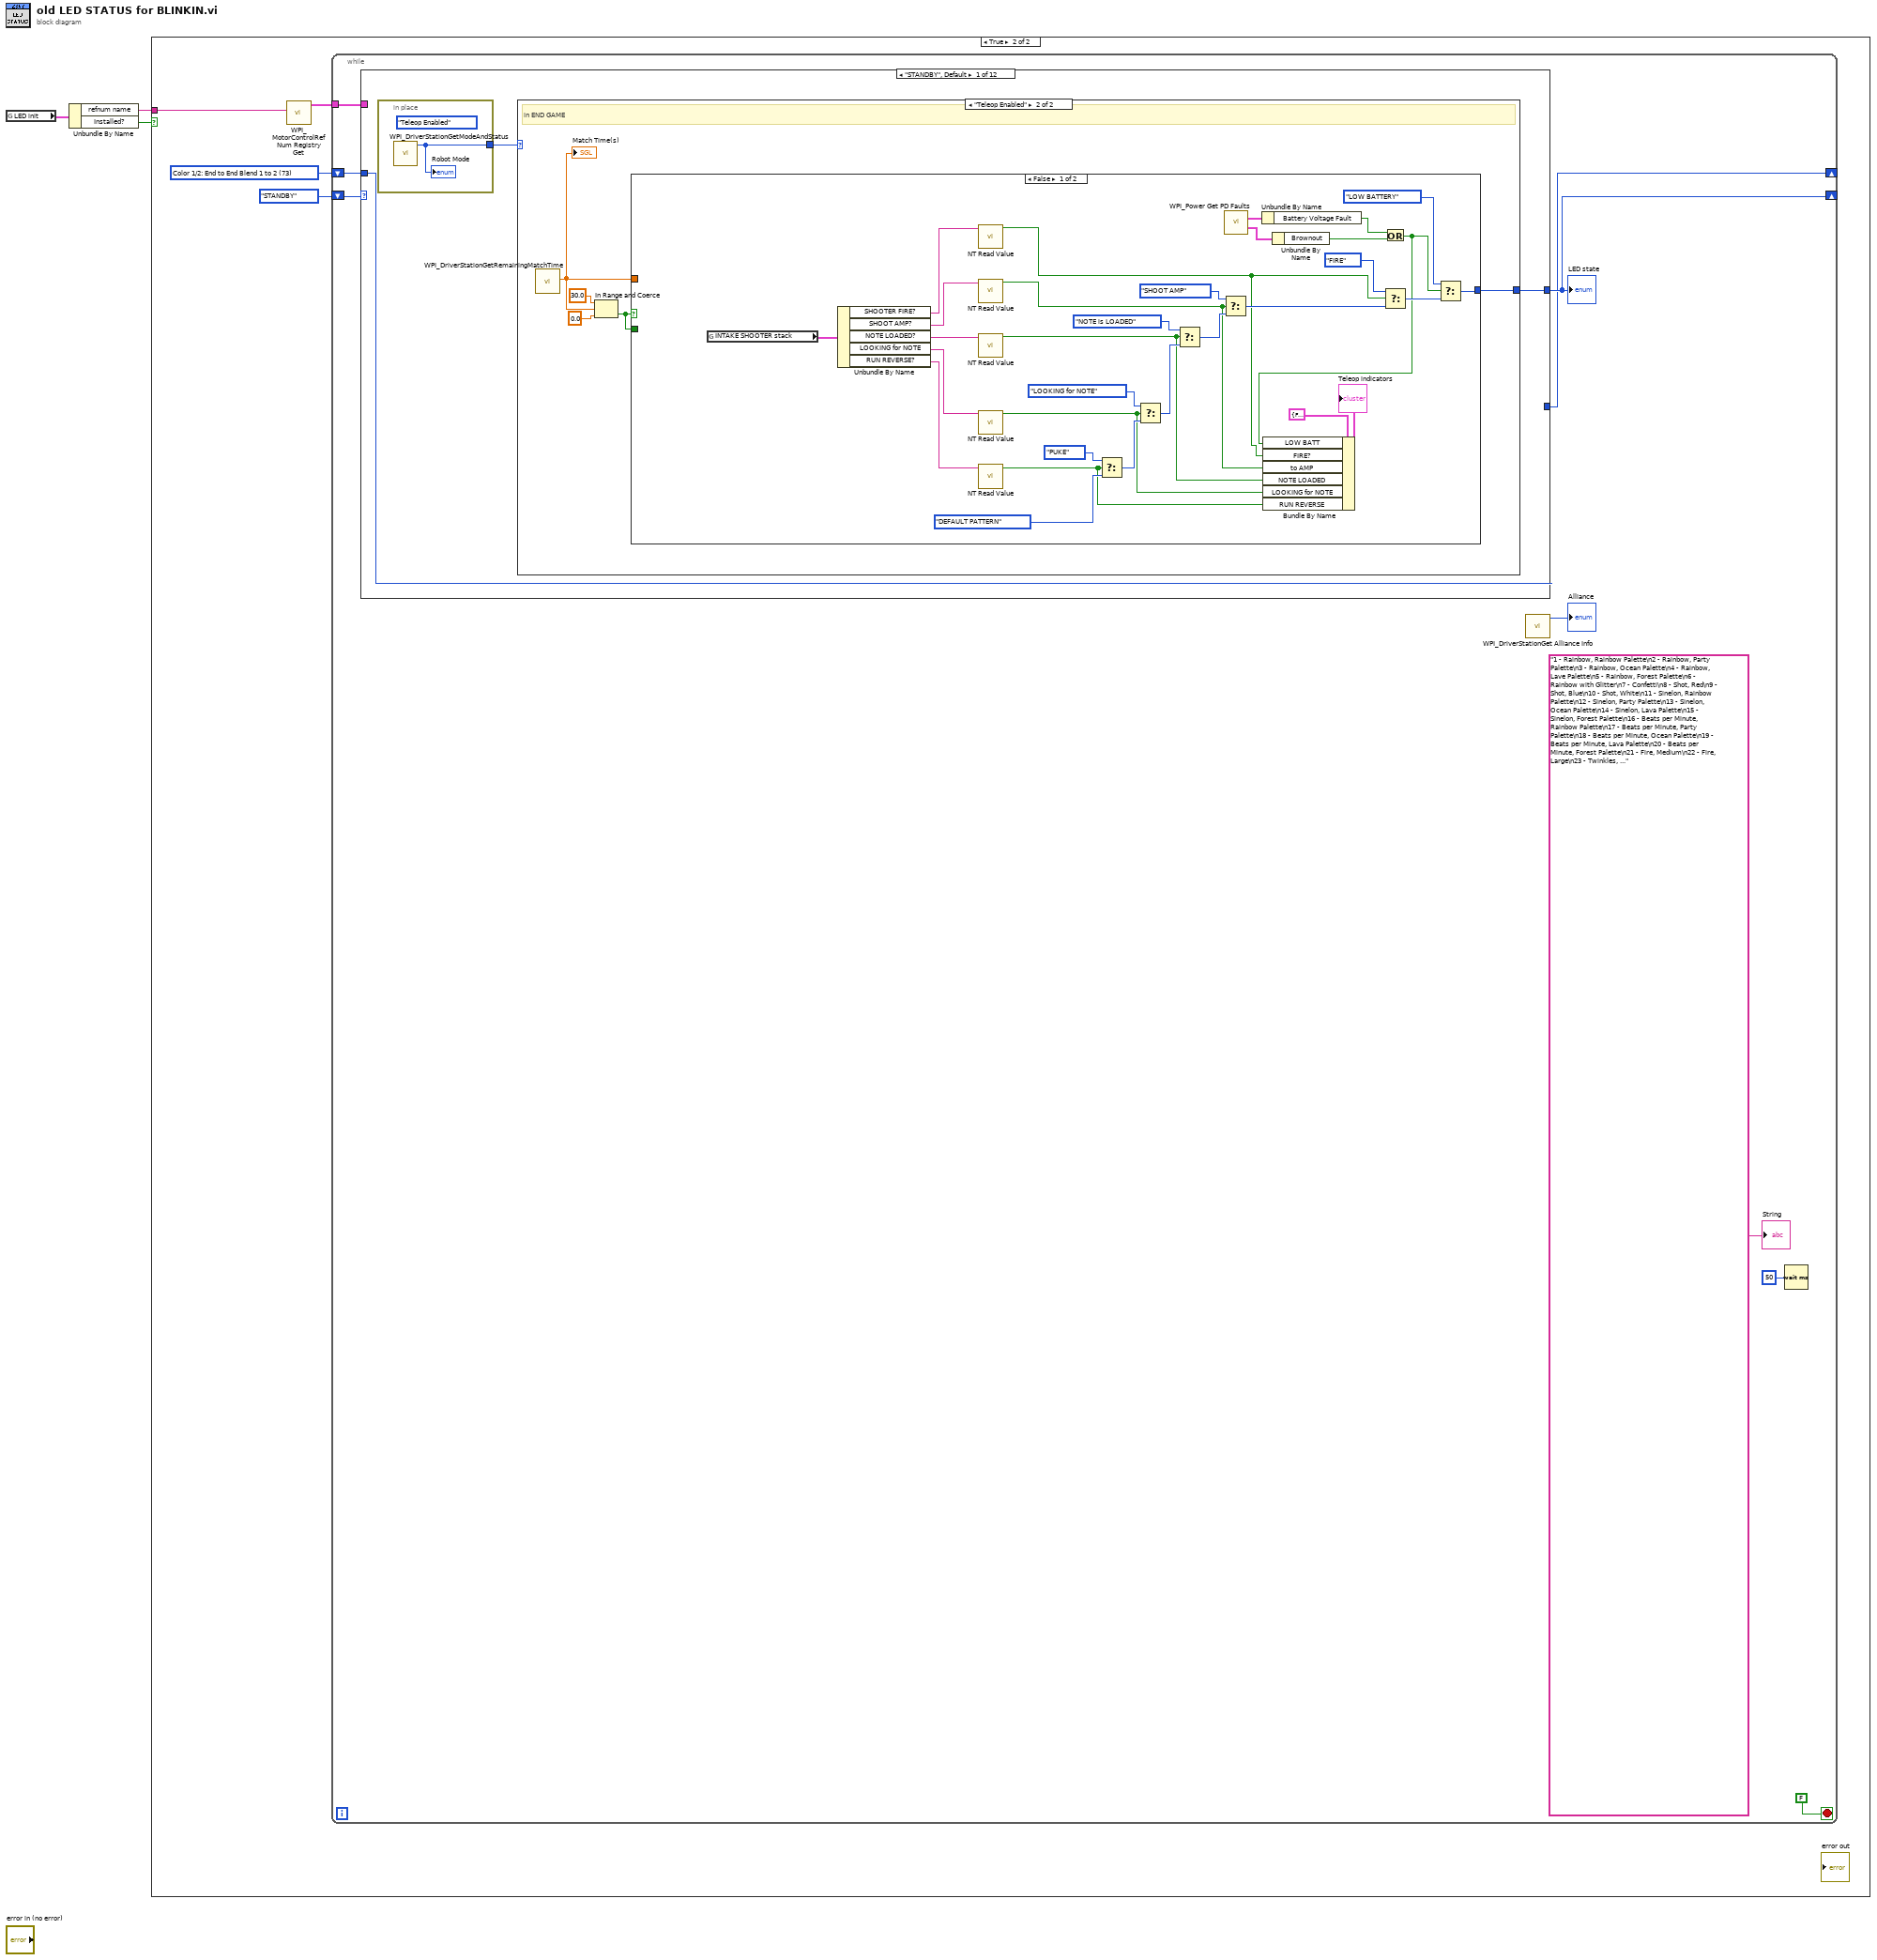
[diagram p0: block diagram]
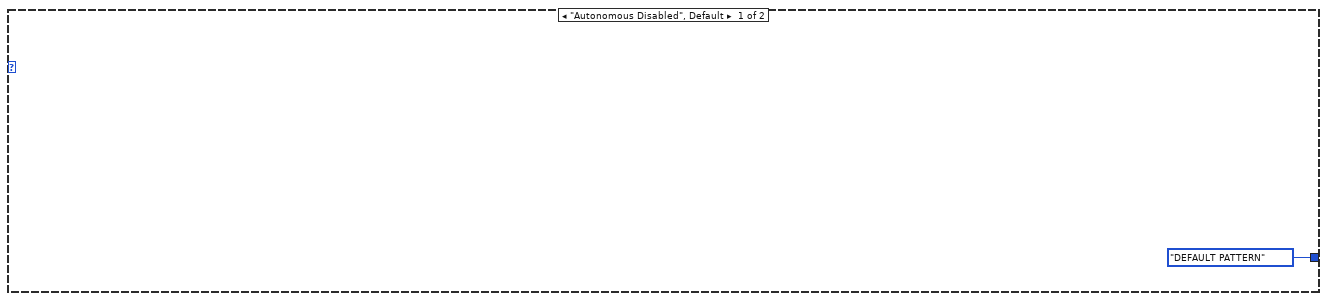
[diagram p3: hidden frame]
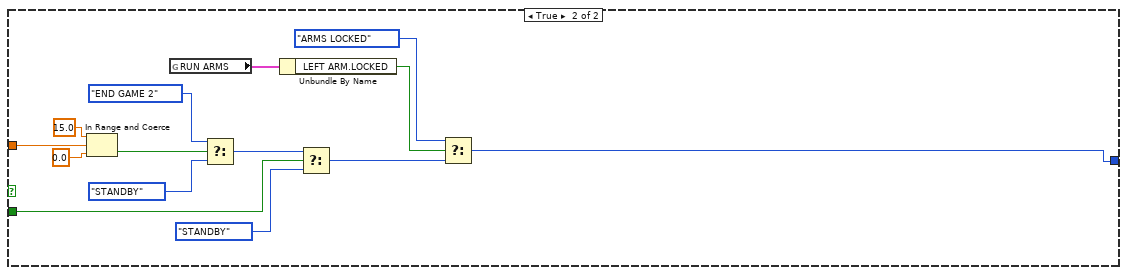
[diagram p4: hidden frame]
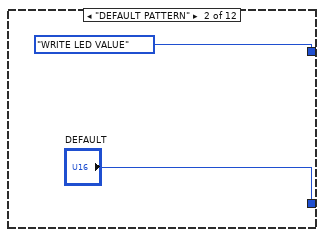
[diagram p5: hidden frame]
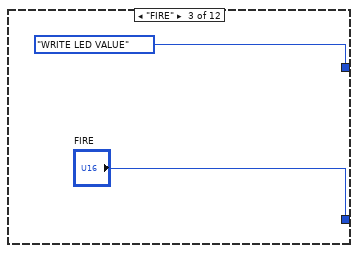
[diagram p6: hidden frame]
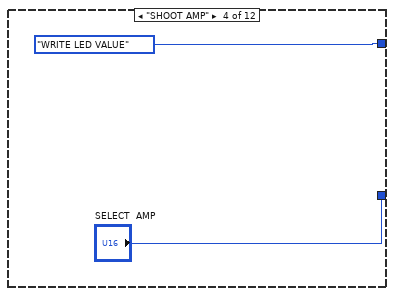
[diagram p7: hidden frame]
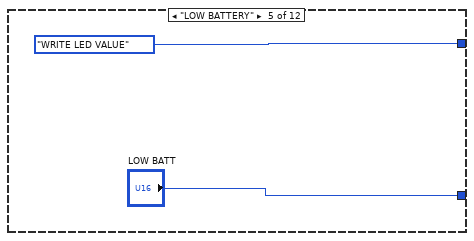
[diagram p8: hidden frame]
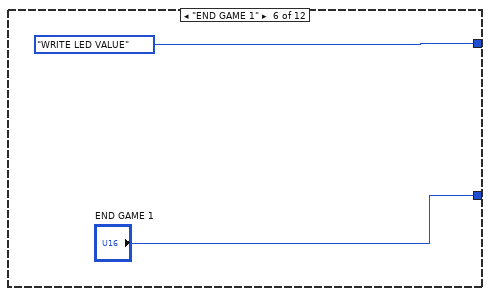
[diagram p9: hidden frame]
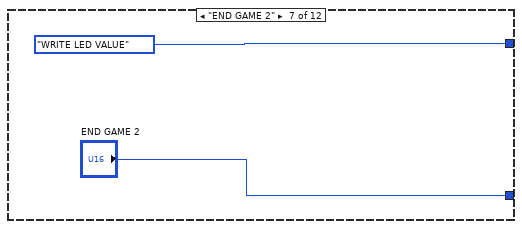
[diagram p10: hidden frame]
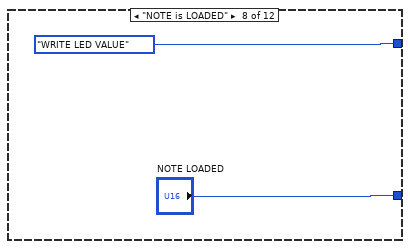
[diagram p11: hidden frame]
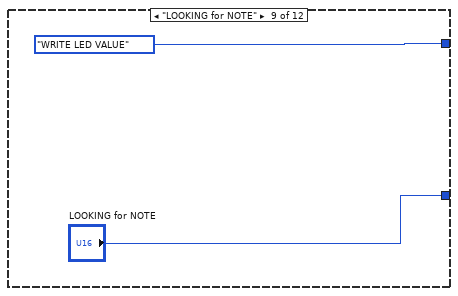
[diagram p12: hidden frame]
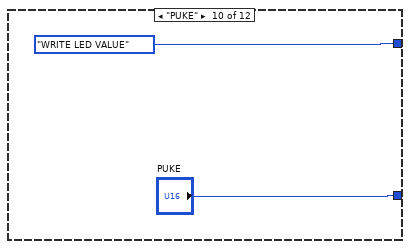
[diagram p13: hidden frame]
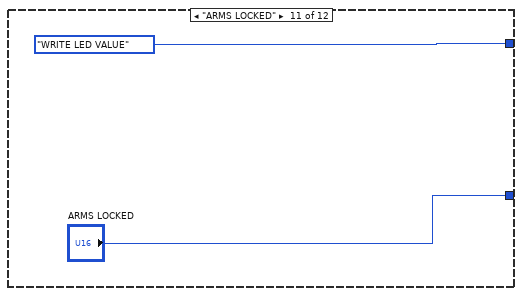
[diagram p14: hidden frame]
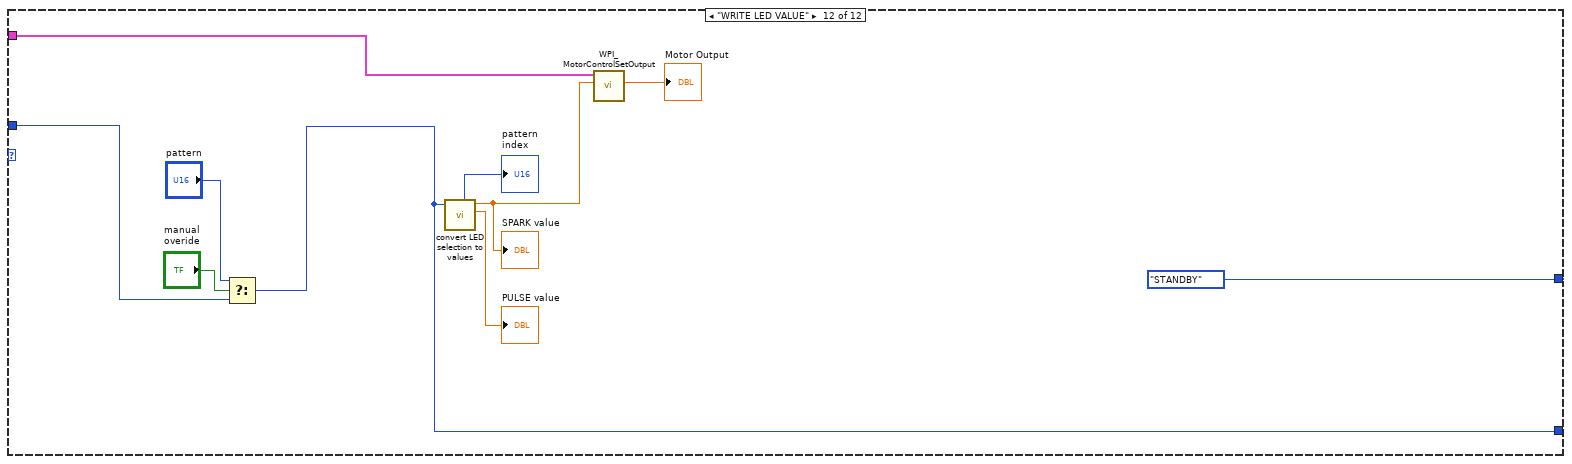
[diagram p15: hidden frame]
diagram:
  n1 = global read "Global INIT.vi" "LED init"() -> (w2:T6)
  n2 = Unbundle By Name(w2) -> ("refnum name"=w1:string, "Installed?"=w3:bool)
  n3 = case shown="True" w3 {
    tunnel: w1 -> [_ w5]
    frame False {
    }
    frame True {
      w6 = T1 73 items=["<<Select a pattern>>", "Rainbow, Rainbow palette", "Rainbow, Party palette", "Rainbow, Ocean palette", "Rainbow, Lava palette", "Rainbow, Forest palette", "Rainbow with glitter", "Confetti", "Shot, Red", "Shot, Blue", "Shot, White", "Sinelon, Rainbow palette", "Sinelon, Party palette", "Sinelon, Ocean palette", "Sinelon, Lava palette", "Sinelon, Forest palette", "BPM, Rainbow palette", "BPM, Party palette", "BPM, Ocean palette", "BPM, Lava palette", "BPM, Forest palette", "Fire, Medium", "Fire, Large", "Twinkles, Rainbow palette", "Twinkles, Party palette", "Twinkles, Ocean palette", "Twinkles, Lava palette", "Twinkles, Forest palette", "Color Waves, Rainbow palette", "Color Waves, Party palette", "Color Waves, Ocean palette", "Color Waves, Lava palette", "Color Waves, Forest palette", "Larson Scanner, Red", "Larson Scanner, Gray", "Light Chase, Red", "Light Chase, Blue", "Light Chase, Gray", "Heartbeat, Red", "Heartbeat, Blue", "Heartbeat, White", "Heartbeat, Gray", "Breath, Red", "Breath, Blue", "Breath, Gray", "Strobe, Red", "Strobe, Blue", "Strobe, Gold", "Strobe, White", "Color 1: End to End Blend to Black", "Color 1: Larson Scanner", "Color 1: Light Chase", "Color 1: Heartbeat Slow", "Color 1: Heartbeat Medium", "Color 1: Heartbeat Fast", "Color 1: Breath Slow", "Color 1: Breath Fast", "Color 1: Shot", "Color 1: Strobe", "Color 2: End to End Blend to Black", "Color 2: Larson Scanner", "Color 2: Light Chase", "Color 2: Heartbeat Slow", "Color 2: Heartbeat Medium", "Color 2: Heartbeat Fast", "Color 2: Breath Slow", "Color 2: Breath Fast", "Color 2: Shot", "Color 2: Strobe", "Color 1/2: Sparkle, 1 on 2", "Color 1/2: Sparkle 2 on 1", "Color 1/2: Gradient", "Color 1/2: BPM", "Color 1/2: End to End Blend 1 to 2", "Color 1/2: End to End Blend 2 to 1", "Color 1/2: setup pattern", "Color 1/2: Twinkles", "Color 1/2: Color Waves", "Color 1/2: Sinelon", "Solid Hot Pink", "Solid Dark Red", "Solid Red", "Solid Red Orange", "Solid Orange", "Solid Gold", "Solid Yellow", "Solid Lawn Green", "Solid Lime", "Solid Dark Green", "Solid Green", "Solid Blue Green", "Solid Aqua", "Solid Sky Blue", "Solid Dark Blue", "Solid Blue", "Solid Blue Violet", "Solid Violet", "Solid White", "Solid Gray", "Solid Dark Gray", "Solid Black"] ("pattern")
      n4 = call <vilib>:"WPI_MotorControlRefNum Registry Get.vi"("refnum name"=w5) -> ("MotorControlDevRef"=w4:T9)  [unwired: 9 in, 1 out]
      n5 = while {
        shift-right: [w14] -> _
        shift-left: ctrl_LED_STATES."STANDBY" -> [w10]
        shift-right: [w8] -> _
        shift-left: w6 -> [w13]
        tunnel: w4 -> [w12]
        stop <- FALSE stop-if-true
        n6 = case shown="\"STANDBY\", Default" w10 {
          tunnel: [w18 ctrl_LED_STATES."WRITE LED VALUE" ctrl_LED_STATES."WRITE LED VALUE" ctrl_LED_STATES."WRITE LED VALUE" ctrl_LED_STATES."WRITE LED VALUE" ctrl_LED_STATES."WRITE LED VALUE" ctrl_LED_STATES."WRITE LED VALUE" ctrl_LED_STATES."WRITE LED VALUE" ctrl_LED_STATES."WRITE LED VALUE" ctrl_LED_STATES."WRITE LED VALUE" ctrl_LED_STATES."WRITE LED VALUE" ctrl_LED_STATES."STANDBY"] -> w14
          tunnel: [w17 "DEFAULT" "FIRE" "SELECT  AMP" "LOW BATT" "END GAME 1" "END GAME 2" "NOTE LOADED" "LOOKING for NOTE" "PUKE" "ARMS LOCKED" w93] -> w8
          tunnel: w13 -> [w17 _ _ _ _ _ _ _ _ _ _ w92]
          tunnel: w12 -> [_ _ _ _ _ _ _ _ _ _ _ w101]
          frame "STANDBY", Default {
            n7 = in-place {
              in-place-border: [w20] -> w19
              (unwired) WPI_DriverStationRobotMode2."Teleop Enabled" ("Robot Mode")
              n8 = call <vilib>:"WPI_DriverStationGetModeAndStatus.vi"() -> ("Robot Mode"=w20:T4)  [unwired: 10 in, 1 out]
              "Robot Mode" <- w20
            }
            n9 = case shown="\"Teleop Enabled\"" w19 {
              tunnel: [ctrl_LED_STATES."DEFAULT PATTERN" w26] -> w18
              frame "Autonomous Disabled", Default {
              }
              frame "Teleop Enabled" {
                # "in END GAME"
                n10 = call <vilib>:"WPI_DriverStationGetRemainingMatchTime.vi"() -> ("Match Time(s)"=w23:sgl)  [unwired: 10 in, 1 out]
                "Match Time(s)" <- w23
                n11 = In Range and Coerce(upper limit=30.0, x=w23, lower limit=0.0) -> (In Range?=w22:bool)  [unwired: 1 out]
                n12 = case shown="False" w22 {
                  tunnel: [w39 w64] -> w26
                  tunnel: w23 -> [_ w62]
                  tunnel: w22 -> [_ w61]
                  frame False {
                    n13 = global read "Global stack names.vi" "INTAKE SHOOTER stack"() -> (w57:T13)
                    n14 = Unbundle By Name(w57) -> ("SHOOTER FIRE?"=w56:string, "SHOOT AMP?"=w55:string, "NOTE LOADED?"=w54:string, "LOOKING for NOTE"=w53:string, "RUN REVERSE?"=w52:string)
                    n15 = call-poly <vilib>:"NT Read Value.vi"("name"=w56) -> ("value"=w31:bool)  [unwired: 8 in, 2 out]
                    n16 = call-poly <vilib>:"NT Read Value.vi"("name"=w55) -> ("value"=w30:bool)  [unwired: 8 in, 2 out]
                    n17 = call-poly <vilib>:"NT Read Value.vi"("name"=w54) -> ("value"=w29:bool)  [unwired: 8 in, 2 out]
                    n18 = call-poly <vilib>:"NT Read Value.vi"("name"=w53) -> ("value"=w28:bool)  [unwired: 8 in, 2 out]
                    n19 = call-poly <vilib>:"NT Read Value.vi"("name"=w52) -> ("value"=w27:bool)  [unwired: 8 in, 2 out]
                    n20 = Select(t=ctrl_LED_STATES."PUKE", s=w27, f=ctrl_LED_STATES."DEFAULT PATTERN") -> (s? t:f=w45:T5)
                    n21 = Select(t=ctrl_LED_STATES."LOOKING for NOTE", s=w28, f=w45) -> (s? t:f=w46:T5)
                    n22 = Select(t=ctrl_LED_STATES."NOTE is LOADED", s=w29, f=w46) -> (s? t:f=w48:T5)
                    n23 = Select(t=ctrl_LED_STATES."SHOOT AMP", s=w30, f=w48) -> (s? t:f=w50:T5)
                    n24 = call <vilib>:"WPI_Power Get PD Faults.vi"() -> ("Faults"=w41:T14, "Sticky Faults"=w40:T15)  [unwired: 12 in, 2 out]
                    n25 = Unbundle By Name(w41) -> ("Battery Voltage Fault"=w37:bool)
                    n26 = Unbundle By Name(w40) -> ("Brownout"=w36:bool)
                    n27 = Or(x=w37, y=w36) -> (x .or. y?=w32:bool)
                    n28 = Bundle By Name(cluster=T2 {"LOW BATT"=FALSE, "FIRE?"=FALSE, "to AMP"=FALSE, "NOTE LOADED"=FALSE, "LOOKING for NOTE"=FALSE, "RUN REVERSE"=FALSE} ("Cluster"), "LOW BATT"=w32, "FIRE?"=w31, "to AMP"=w30, "NOTE LOADED"=w29, "LOOKING for NOTE"=w28, "RUN REVERSE"=w27) -> (→"Teleop indicators":T2)
                    n29 = Select(t=ctrl_LED_STATES."FIRE", s=w31, f=w50) -> (s? t:f=w38:T5)
                    n30 = Select(t=ctrl_LED_STATES."LOW BATTERY", s=w32, f=w38) -> (s? t:f=w39:T5)
                  }
                  frame True {
                    n31 = In Range and Coerce(upper limit=sgl 15.0 ("y"), x=w62, lower limit=sgl 0.0) -> (In Range?=w71:bool)  [unwired: 1 out]
                    n32 = global read "Global odometry.vi" "RUN ARMS"() -> (w63:T16)
                    n33 = Select(t=ctrl_LED_STATES."END GAME 2", s=w71, f=ctrl_LED_STATES."STANDBY") -> (s? t:f=w60:T5)
                    n34 = Unbundle By Name(w63) -> ("LEFT ARM.LOCKED"=w67:bool)
                    n35 = Select(t=w60, s=w61, f=ctrl_LED_STATES."STANDBY") -> (s? t:f=w59:T5)
                    n36 = Select(t=ctrl_LED_STATES."ARMS LOCKED", s=w67, f=w59) -> (s? t:f=w64:T5)
                  }
                }
              }
            }
          }
          frame "DEFAULT PATTERN" {
          }
          frame "FIRE" {
          }
          frame "SHOOT AMP" {
          }
          frame "LOW BATTERY" {
          }
          frame "END GAME 1" {
          }
          frame "END GAME 2" {
          }
          frame "NOTE is LOADED" {
          }
          frame "LOOKING for NOTE" {
          }
          frame "PUKE" {
          }
          frame "ARMS LOCKED" {
          }
          frame "WRITE LED VALUE" {
            n37 = Select(t="pattern", s="manual\noveride", f=w92) -> (s? t:f=w93:T1)
            n38 = call "convert LED selection to values.vi"("Blinkin LED pattern"=w93) -> ("PULSE value"=→"PULSE value":dbl, "SPARK value"=w100:dbl, "pattern\nindex"=→"pattern\nindex":u16)  [unwired: 8 in]
            "SPARK value" <- w100
            n39 = call <vilib>:"WPI_MotorControlSetOutput.vi"("Output"=w100, "MotorControlDevRef"=w101) -> ("Motor Output"=→"Motor Output":dbl)  [unwired: 7 in, 2 out]
          }
        }
        "LED state" <- w14
        n40 = call <vilib>:"WPI_DriverStationGet Alliance Info.vi"() -> ("Alliance"=→"Alliance":T3)  [unwired: 6 in, 5 out]
        n41 = Wait (ms)(milliseconds to wait=u32 50) -> ()  [unwired: 1 out]
        "String" <- "1 - Rainbow, Rainbow Palette\n2 - Rainbow, Party Palette\n3 - Rainbow, Ocean Palette\n4 - Rainbow, Lave Palette\n5 - Rainbow, Forest Palette\n6 - Rainbow with Glitter\n7 - Confetti\n8 - Shot, Red\n9 - Shot, Blue\n10 - Shot, White\n11 - Sinelon, Rainbow Palette\n12 - Sinelon, Party Palette\n13 - Sinelon, Ocean Palette\n14 - Sinelon, Lava Palette\n15 - Sinelon, Forest Palette\n16 - Beats per Minute, Rainbow Palette\n17 - Beats per Minute, Party Palette\n18 - Beats per Minute, Ocean Palette\n19 - Beats per Minute, Lava Palette\n20 - Beats per Minute, Forest Palette\n21 - Fire, Medium\n22 - Fire, Large\n23 - Twinkles, Rainbow Palette\n24 - Twinkles, Party Palette\n25 - Twinkles, Ocean Palette\n26 - Twinkles, Lava Palette\n27 - Twinkles, Forest Palette\n28 - Color Waves, Rainbow Palette\n29 - Color Waves, Party Palette\n30 - Color Waves, Ocean Palette\n31 - Color Waves, Lava Palette\n32 - Color Waves, Forest Palette\n33 - Larson Scanner, Red\n34 - Larson Scanner, Gray\n35 - Light Chase, Red\n36 - Light Chase, Blue\n37 - Light Chase, Gray\n38 - Heartbeat, Red\n39 - Heartbeat, Blue\n40 - Heartbeat, White\n41 - Heartbeat, Gray\n42 - Breath, Red\n43 - Breath, Blue\n44 - Breath, Gray\n45 - Strobe, Red\n46 - Strobe, Blue\n47 - Strobe, Gold\n48 - Strobe, White\n49 - Color 1: End to End Blend to Black\n50 - Color 1: Larson Scanner\n51 - Color 1: Light Chase\n52 - Color 1: Heartbeat Slow\n53 - Color 1: Heartbeat Medium\n54 - Color 1: Heartbeat Fast\n55 - Color 1: Breath Slow\n56 - Color 1: Breath Fast\n57 - Color 1: Shot\n58 - Color 1: Strobe\n59 - Color 2: End to End Blend to Black\n60 - Color 2: Larson Scanner\n61 - Color 2: Light Chase\n62 - Color 2: Heartbeat Slow\n63 - Color 2: Heartbeat Medium\n64 - Color 2: Heartbeat Fast\n65 - Color 2: Breath Slow\n66 - Color 2: Breath Fast\n67 - Color 2: Shot\n68 - Color 2: Strobe\n69 - Color 1/2: Sparkle, Color 1 on Color 2\n70 - Color 1/2: Sparkle, Color 2 on Color 1\n71 - Color 1/2: Color Gradient, Color 1 and 2\n72 - Color 1/2: Beats per Minute, Color 1 and 2\n73 - Color 1/2: End to End Blend, Color 1 to 2\n74 - Color 1/2: End to End Blend\n75 - Color 1/2:  no blending (Setup Pattern)\n76 - Color 1/2: Twinkles\n77 - Color 1/2: Color Waves\n78 - Color 1/2: Sinelon\n79 - Solid Hot Pink\n80 - Solid Dark red\n81 - Solid Red\n82 - Solid Red Orange\n83 - Solid Orange\n84 - Solid Gold\n85 - Solid Yellow\n86 - Solid Lawn Green\n87 - Solid Lime\n88 - Solid Dark Green\n89 - Solid Green\n90 - Solid Blue Green\n91 - Solid Aqua\n92 - Solid Sky Blue\n93 - Solid Dark Blue\n94 - Solid Blue\n95 - Solid Blue Violet\n96 - Solid Violet\n97 - Solid White\n98 - Solid Gray\n99 - Solid Dark Gray\n100 - Solid Black\n" ("String")
      }
    }
  }
